vi "DLPConfigurationXMLNew-Write.vi"() -> ()   [LabVIEW 2022 SP3]
uses:
  Controls/DLPPrinterInitXML.ctl
  Classes/DLP2/DataTypes/DLP2_PrinterCompensationProperties.ctl
  Classes/DLP2/DataTypes/DLP2_PrinterHeadProperties.ctl
  Controls/DLPConfig)Init_HeadPropertyAttr--Cluster.ctl
panel:
  out "XML File Path (duplicate)":path
  in  "XML File Path":path
  in  "DLP":T1
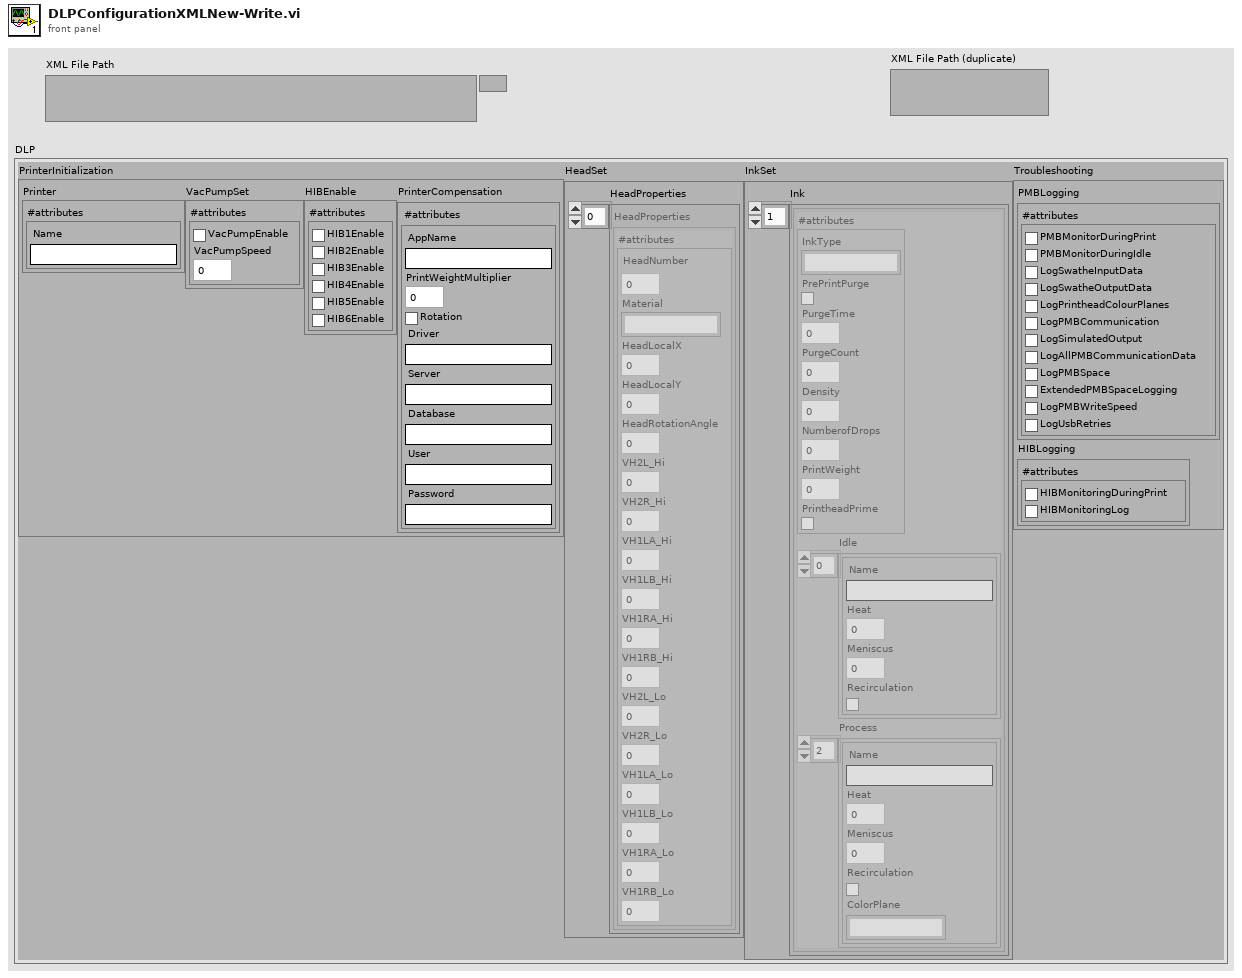
[diagram p1: front panel]
types:
  T1 = typedef "DLPPrinterInitXML.ctl" = cluster{"PrinterInitialization":cluster{"Printer":cluster{"#attributes":cluster{"Name":string}}, "VacPumpSet":cluster{"#attributes":cluster{"VacPumpEnable":bool, "VacPumpSpeed":dbl}}, "HIBEnable":cluster{"#attributes":cluster{"HIB1Enable":bool, "HIB2Enable":bool, "HIB3Enable":bool, "HIB4Enable":bool, "HIB5Enable":bool, "HIB6Enable":bool}}, "PrinterCompensation":T2}, "HeadSet":cluster{"HeadProperties":T3[]}, "InkSet":cluster{"Ink":cluster{"#attributes":cluster{"InkType":string, "PrePrintPurge":bool, "PurgeTime":dbl, "PurgeCount":i32, "Density":dbl, "NumberofDrops":i32, "PrintWeight":dbl, "PrintheadPrime":bool}, "Idle":cluster{"Name":string, "Heat":dbl, "Meniscus":dbl, "Recirculation":bool}[], "Process":cluster{"Name":string, "Heat":dbl, "Meniscus":dbl, "Recirculation":bool, "ColorPlane":string}[]}[]}, "Troubleshooting":cluster{"PMBLogging":cluster{"#attributes":cluster{"PMBMonitorDuringPrint":bool, "PMBMonitorDuringIdle":bool, "LogSwatheInputData":bool, "LogSwatheOutputData":bool, "LogPrintheadColourPlanes":bool, "LogPMBCommunication":bool, "LogSimulatedOutput":bool, "LogAllPMBCommunicationData":bool, "LogPMBSpace":bool, "ExtendedPMBSpaceLogging":bool, "LogPMBWriteSpeed":bool, "LogUsbRetries":bool}}, "HIBLogging":cluster{"#attributes":cluster{"HIBMonitoringDuringPrint":bool, "HIBMonitoringLog":bool}}}}
  T2 = typedef "DLP2_PrinterCompensationProperties.ctl" = cluster{"#attributes":cluster{"AppName":string, "PrintWeightMultiplier":dbl, "Rotation":bool, "Driver":string, "Server":string, "Database":string, "User":string, "Password":string}}
  T3 = typedef "DLP2_PrinterHeadProperties.ctl" = cluster{"#attributes":T4}
  T4 = typedef "DLPConfig)Init_HeadPropertyAttr--Cluster.ctl" = cluster{"HeadNumber":u8, "Material":string, "HeadLocalX":dbl, "HeadLocalY":dbl, "HeadRotationAngle":dbl, "VH2L_Hi":dbl, "VH2R_Hi":dbl, "VH1LA_Hi":dbl, "VH1LB_Hi":dbl, "VH1RA_Hi":dbl, "VH1RB_Hi":dbl, "VH2L_Lo":dbl, "VH2R_Lo":dbl, "VH1LA_Lo":dbl, "VH1LB_Lo":dbl, "VH1RA_Lo":dbl, "VH1RB_Lo":dbl}
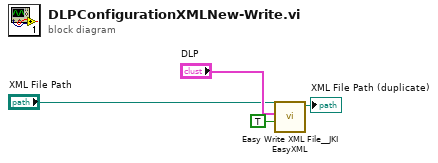
[diagram p0: block diagram]
diagram:
  n1 = call <vilib>:"Easy Write XML File__JKI EasyXML.vi"("Overwrite File? (false)"=TRUE, "LabVIEW Data"="DLP", "XML File Path"="XML File Path") -> ("XML File Path (duplicate)"=→"XML File Path (duplicate)":path)  [unwired: 7 in, 1 out]
